vi "Example Advanced.vi"() -> ()   [LabVIEW 2014]
doc: "This examples shows off many of the basic usage patterns of the datagrid."
uses:
  System.Windows.Forms
  GridColumn/ColumnDefinition.ctl
  GridColumn/ColumnType.ctl
  DataGridView/DataGridView.lvclass
  DataGrid.lvlib
  DataTable/DataTable.lvclass
  GridColumn/GridColumn.lvclass
panel:
  in  "Remove":bool
  in  "#AddRows":i32=15
  in  "Add":bool
  in  "Disabled State Cell 1, 5":T1(ring)
  out "Events":string
  in  "# of Rows":i32=15
  in  "ColumnSetup":T2[](array[typedef])=[{"name"="Text", "caption"="Text", "datatype"=enum."string", "Params"="", "AutoSizeMode"=16, "FillWeight"=15.0, "MinWidth"=40}, {"name"="Details", "caption"="Text", "datatype"=enum."string", "Params"="", "AutoSizeMode"=16, "FillWeight"=85.0, "MinWidth"=150}, {"name"="Time", "caption"="", "datatype"=enum."timestamp", "Params"="", "AutoSizeMode"=1, "FillWeight"=1.0, "MinWidth"=120}, {"name"="Selection", "caption"="", "datatype"=enum."combo", "Params"="One|Two|Three", "AutoSizeMode"=6, "FillWeight"=1.0, "MinWidth"=80}, {"name"="Function", "caption"="", "datatype"=enum."button", "Params"="", "AutoSizeMode"=6, "FillWeight"=1.0, "MinWidth"=50}, {"name"="Value", "caption"="", "datatype"=enum."numeric", "Params"="", "AutoSizeMode"=6, "FillWeight"=1.0, "MinWidth"=10}, {"name"="Active", "caption"="", "datatype"=enum."check", "Params"="", "AutoSizeMode"=6, "FillWeight"=1.0, "MinWidth"=10}, {"name"="Status", "caption"="", "datatype"=enum."image", "Params"="", "AutoSizeMode"=6, "FillWeight"=1.0, "MinWidth"=10}, {"name"="Link", "caption"="", "datatype"=enum."link", "Params"="", "AutoSizeMode"=1, "FillWeight"=100.0, "MinWidth"=50}] {"MinWidth" min=2 step=1; "AutoSizeMode" items=["None"=1, "ColumnHeader"=2, "AllCellsExceptHeader"=4, "AllCells"=6, "DisplayedCellsExceptHeader"=8, "DisplayedCells"=10, "Fill"=16]; "FillWeight" min=1 max=100}
  in  "DataGridView":refnum<k24>(container)
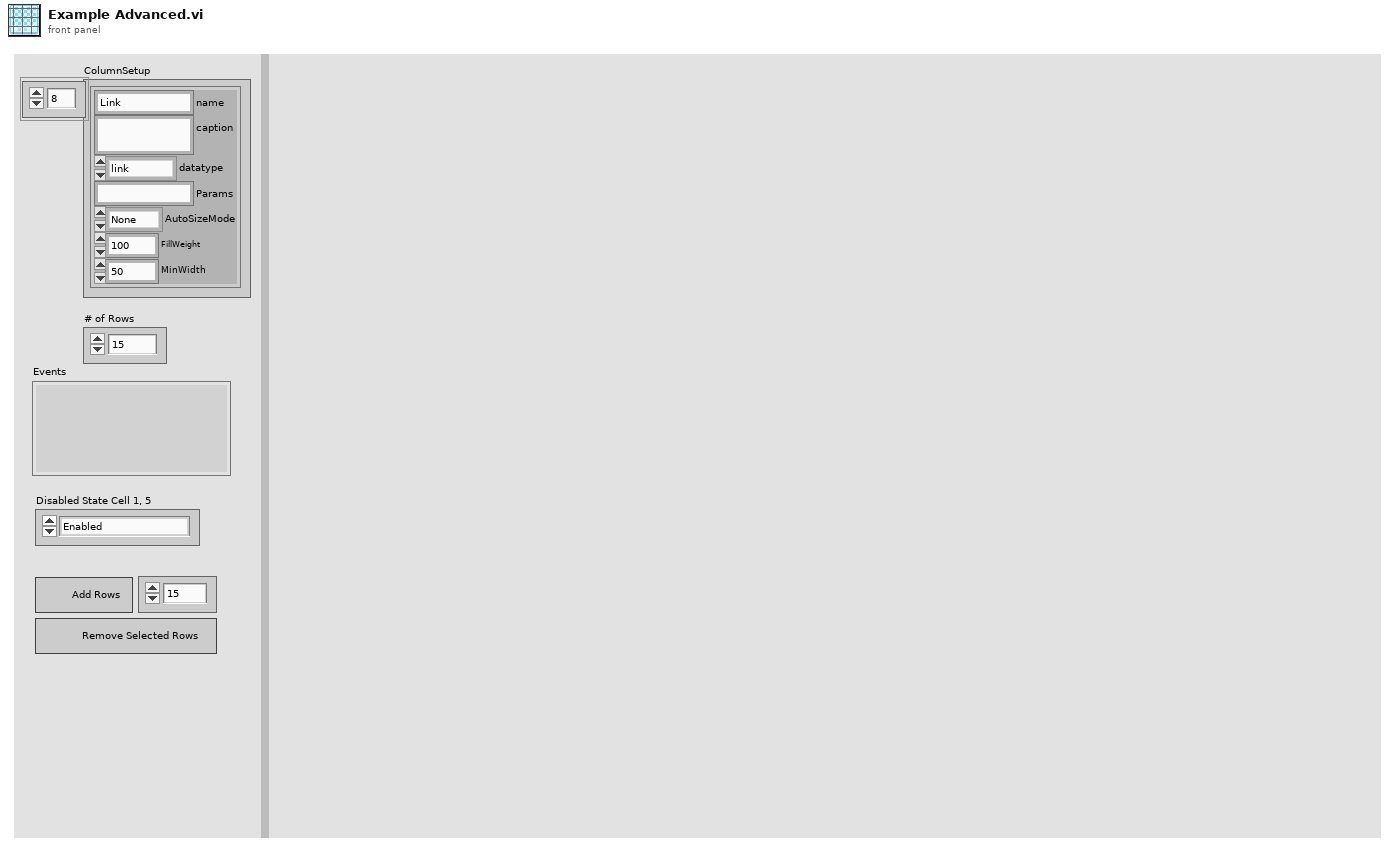
[diagram p1: front panel]
types:
  T1 = enum8{"Enabled", "Disabled", "Disabled and Grayed Out"}
  T2 = typedef "DataGrid.lvlib/GridColumn.lvclass/ColumnDefinition.ctl" = cluster{"name":string, "caption":string, "datatype":T3, "Params":string, "AutoSizeMode":i32, "FillWeight":sgl, "MinWidth":u32}
  T3 = typedef "DataGrid.lvlib/GridColumn.lvclass/ColumnType.ctl" = enum16{"string", "image", "check", "numeric", "timestamp", "button", "combo", "link"}
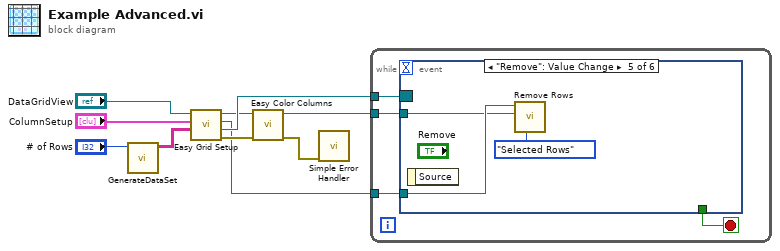
[diagram p0: block diagram]
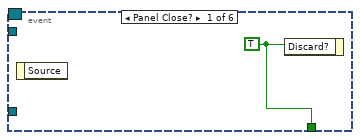
[diagram p2: hidden frame]
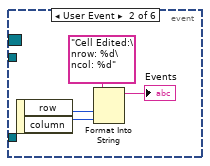
[diagram p3: hidden frame]
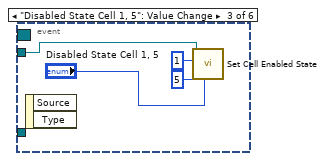
[diagram p4: hidden frame]
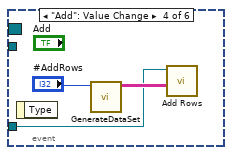
[diagram p5: hidden frame]
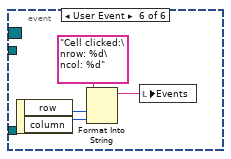
[diagram p6: hidden frame]
diagram:
  n1 = call "GenerateDataSet.vi"("Records"="# of Rows") -> ("DataGrid"=w7:string[][])  [unwired: 10 in]
  n2 = call "Easy Grid Setup.vi"("DataSource Data"=w7, "ColumnSetup"="ColumnSetup", ".net datagridview ref"="DataGridView") -> ("error out"=w5:errorcluster, "Grid RegisteredEvents"=w6:refnum<event-registration>, "DataTable out"=w1:refnum<class "DataTable.lvclass">, "DataGrid out"=w3:refnum<class "DataGridView.lvclass">)  [unwired: 5 in]
  n3 = call "Easy Color Columns.vi"("error in (no error)"=w5, "DataGridView in"=w3) -> ("error out"=w4:errorcluster, "DataGridView out"=w2:refnum<class "DataGridView.lvclass">)  [unwired: 8 in]
  n4 = call <vilib>:"Simple Error Handler.vi"("error in (no error)"=w4) -> ()  [unwired: 4 in, 5 out]
  n5 = while {
    tunnel: w6 -> [w13]
    tunnel: w2 -> [w12]
    tunnel: w1 -> [w11]
    stop <- w14 stop-if-true
    n6 = event shown="[4] \"Remove\": Value Change" {
      selector: w13 -> [_ _ _ _ _ _]
      dyn-events: _ -> [_ _ _ _ _ _]
      timeout: _ -> [_ _ _ _ _ _]
      tunnel: [w15 _ _ _ _ _] -> w14
      tunnel: w12 -> [_ _ w20 _ w28 _]
      tunnel: w11 -> [_ _ _ w24 w29 _]
      event Panel Close? {
        w15 = TRUE ("Discard?")
        n7 = event-data() -> ()  [unwired: 1 in, 1 out]
        n8 = event-data("Discard?"=w15) -> ()  [unwired: 1 in, 1 out]
      }
      event User Event {
        n9 = event-data() -> ("row"=w17:i32, "column"=w18:i32)  [unwired: 1 in]
        n10 = Format Into String(format string="Cell Edited:\nrow: %d\ncol: %d" ("message"), w17, w18) -> (resulting string=→"Events":string)  [unwired: 2 in, 1 out]
      }
      event "Disabled State Cell 1, 5": Value Change {
        n11 = event-data() -> ()  [unwired: 1 in, 2 out]
        n12 = call "Set Cell Enabled State.vi"("Disabled State"="Disabled State Cell 1, 5", "rowIndex"=5, "colindex"=1, "DataGridView in"=w20) -> ()  [unwired: 6 in, 2 out]
      }
      event "Add": Value Change {
        n13 = event-data() -> ()  [unwired: 1 in, 1 out]
        n14 = call "GenerateDataSet.vi"("Records"="#AddRows") -> ("DataGrid"=w25:string[][])  [unwired: 10 in]
        n15 = call "Add Rows.vi"("String Data"=w25, "DataTable in"=w24) -> ()  [unwired: 8 in, 2 out]
      }
      event "Remove": Value Change {
        n16 = event-data() -> ()  [unwired: 1 in, 1 out]
        n17 = call "Remove Rows.vi"("Mode"=enum16{"Selected Rows", "Input Rows"}."Selected Rows", "DataGridView in"=w28, "DataTable in"=w29) -> ()  [unwired: 8 in, 1 out]
      }
      event User Event {
        n18 = event-data() -> ("row"=w31:i32, "column"=w32:i32)  [unwired: 1 in]
        n19 = Format Into String(format string="Cell clicked:\nrow: %d\ncol: %d" ("message"), w31, w32) -> (resulting string=w30:string)  [unwired: 2 in, 1 out]
        n20 = local write "Events"(w30) -> ()
      }
    }
  }
